vi "Flock_RetrieveFIRSTdata_Process.vi"(11 "Process":string) -> ()   [LabVIEW 2013, in "Flock_RetrieveFIRSTdata.lvlib"]
uses:
  Flock_RetrieveFIRSTdata.lvlib
  Shared Code/AMC/VI Source/LocalProcessMessaging/Flock_Shared_LocalProcessMessaging.lvlib
  Shared Code/AMC/VI Source/CentralProcessMessaging/Flock_Shared_CentralProcessMessaging.lvlib
  Shared Code/AMC/VI Source/Error Handling/Flock_ErrorHandling.lvlib
panel:
  in  "Stand Alone?":bool
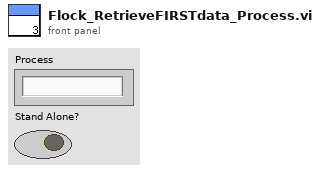
[diagram p1: front panel]
types:
  T1 = typedef "Flock_Shared_Messaging.lvlib/ProcessList.ctl" = string
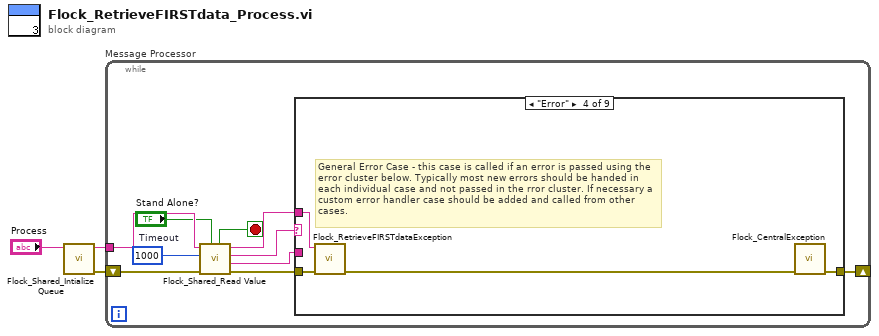
[diagram p0: block diagram]
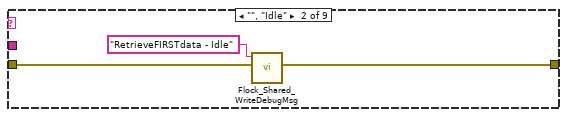
[diagram p3: hidden frame]
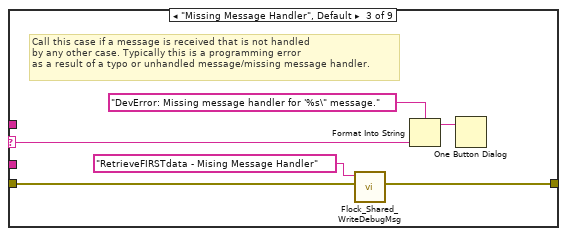
[diagram p4: hidden frame]
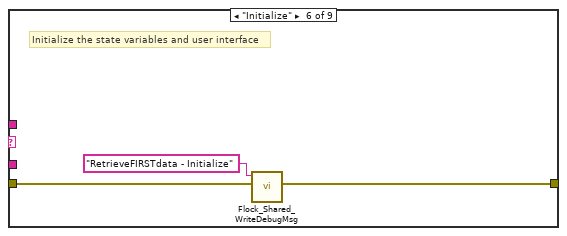
[diagram p6: hidden frame]
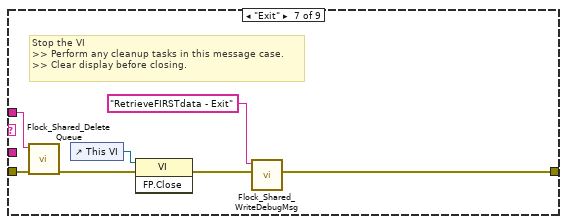
[diagram p7: hidden frame]
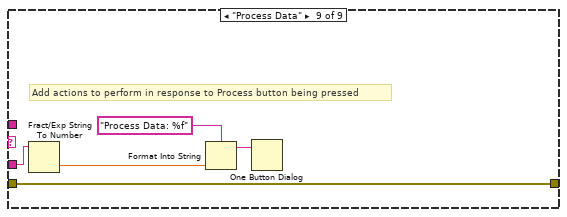
[diagram p9: hidden frame]
diagram:
  n1 = call "Flock_Shared_Intialize Queue.vi"("Enum"="Process") -> ("error out"=w2:errorcluster, "Process Name"=w1:T1)  [unwired: 9 in]
  n2 = while "Message Processor" {
    shift-left: w2 -> [w11]
    shift-right: [w13] -> _
    tunnel: w1 -> [w6]
    stop <- w7 stop-if-true
    w12 = 1000  # Timeout
    n3 = call "Flock_Shared_Read Value.vi"("Stand Alone?"="Stand Alone?", "error in (no error)"=w11, "timeout (1ms)"=w12, "Process"=w6) -> ("error out"=w10:errorcluster, "Message Value"=w8:string, "Message Name"=w9:string, "Process"=w5:T1, "Exit Process"=w7:bool)  [unwired: 3 in]
    n4 = case shown="\"Error\"" w9 {
      selector: w9 -> [_ _ w23 _ _ _ _ _ _]
      tunnel: [w14 w15 w19 w25 w28 w30 w33 w39 w41] -> w13
      tunnel: w10 -> [w14 w16 w20 w27 w28 w31 w38 w39 w41]
      tunnel: w8 -> [_ _ _ _ _ _ _ _ w40]
      tunnel: w5 -> [_ _ _ w24 _ _ w37 _ _]
      frame "---------- Framework Operations ----------" {
        # "Dummy case to add a seperator in the Case Structure menu"
      }
      frame "", "Idle" {
        n5 = call "Flock_Shared_WriteDebugMsg.vi"("error in (no error)"=w16, "Current Message Case"="RetrieveFIRSTdata - Idle") -> ("error out"=w15:errorcluster)  [unwired: 9 in]
      }
      frame "Missing Message Handler", Default {
        # "Call this case if a message is received that is not handled \nby any other case. Typically this is a programming error\nas a result of a typo or unhandled message/missing message handler."
        n6 = call "Flock_Shared_WriteDebugMsg.vi"("error in (no error)"=w20, "Current Message Case"="RetrieveFIRSTdata - Mising Message Handler") -> ("error out"=w19:errorcluster)  [unwired: 9 in]
        n7 = Format Into String(format string="DevError: Missing message handler for '%s\" message." ("message"), w23) -> (resulting string=w21:string)  [unwired: 2 in, 1 out]
        n8 = One Button Dialog(message=w21) -> ()  [unwired: 2 out]
      }
      frame "Error" {
        # "General Error Case - this case is called if an error is passed using the error cluster below. Typically most new errors should be handed in each individual case and not passed in the rror cluster. If necessary a custom error handler case should be added and called from other cases."
        n9 = call "Flock_RetrieveFIRSTdataException.vi"("Error In"=w27, "Process List"=w24) -> ("Error Out"=w26:errorcluster)  [unwired: 9 in]
        n10 = call "Flock_CentralException.vi"("Error In"=w26) -> ("Error Out"=w25:errorcluster)  [unwired: 10 in]
      }
      frame "---------- Generic Operations ----------" {
        # "Dummy case to add a seperator in the Case Structure menu"
      }
      frame "Initialize" {
        # "Initialize the state variables and user interface"
        n11 = call "Flock_Shared_WriteDebugMsg.vi"("error in (no error)"=w31, "Current Message Case"="RetrieveFIRSTdata - Initialize") -> ("error out"=w30:errorcluster)  [unwired: 9 in]
      }
      frame "Exit" {
        # "Stop the VI\n>> Perform any cleanup tasks in this message case.\n>> Clear display before closing."
        n12 = call "Flock_Shared_Delete Queue.vi"("Error In"=w38, "Process Name"=w37) -> ("Error Out"=w35:errorcluster)  [unwired: 9 in]
        n13 = control-ref of="This VI"() -> (w36:refnum<vi>)
        n14 = invoke class="VI" method="FP.Close"(reference=w36, error in=w35) -> (error out=w34:errorcluster)  [unwired: 1 in, 2 out]
        n15 = call "Flock_Shared_WriteDebugMsg.vi"("error in (no error)"=w34, "Current Message Case"="RetrieveFIRSTdata - Exit") -> ("error out"=w33:errorcluster)  [unwired: 9 in]
      }
      frame "---------- Application Operations ----------" {
        # "Dummy case to add a seperator in the Case Structure menu"
      }
      frame "Process Data" {
        # "Add actions to perform in response to Process button being pressed"
        n16 = Fract/Exp String To Number(string=w40) -> (number=w44:dbl)  [unwired: 4 out]
        n17 = Format Into String(format string="Process Data: %f" ("message"), w44) -> (resulting string=w42:string)  [unwired: 2 in, 1 out]
        n18 = One Button Dialog(message=w42) -> ()  [unwired: 2 out]
      }
    }
  }
